vi "Matr_lin.vi"(2 "Date":u8, 3 "Linia":u8, 4 "Adresa port paralel":u16) -> (0 "C0-C3":u8, 1 "D0-D7":u8)   [LabVIEW 2009]
uses:
  <vilib>/Platform/portaccess.llb/Out Port8.vi
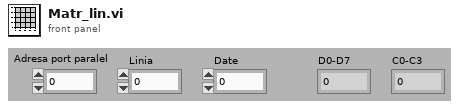
[diagram p1: front panel]
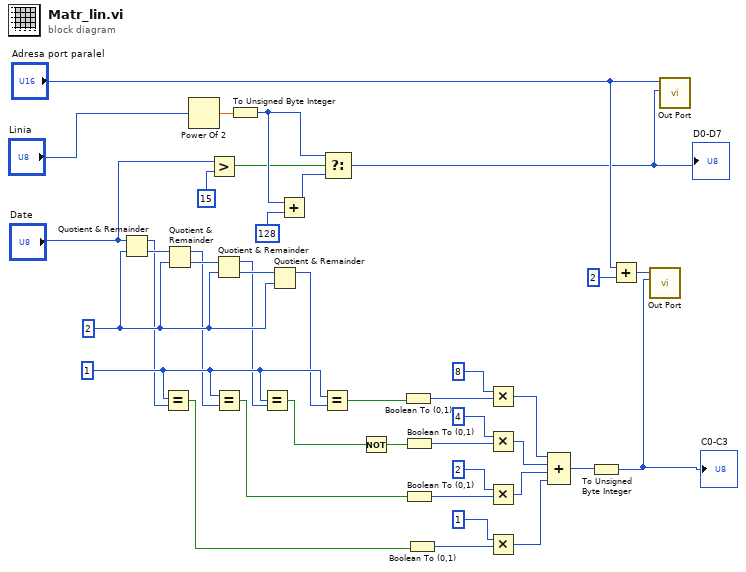
[diagram p0: block diagram]
diagram:
  w19 = 2
  w23 = 1
  n1 = Quotient & Remainder(x="Date", y=w19) -> (x-y*floor(x/y)=w15:i32, floor(x/y)=w22:i32)
  n2 = Equal?(x=w23, y=w15) -> (x = y?=w3:bool)
  n3 = Quotient & Remainder(x=w22, y=w19) -> (x-y*floor(x/y)=w16:i32, floor(x/y)=w21:i32)
  n4 = Power Of 2(x="Linia") -> (2^x=w13:dbl)
  n5 = Greater?(x="Date", y=u8 15) -> (0:w12:bool)
  n6 = Quotient & Remainder(x=w21, y=w19) -> (x-y*floor(x/y)=w17:i32, floor(x/y)=w20:i32)
  n7 = Equal?(x=w23, y=w16) -> (x = y?=w4:bool)
  n8 = To Unsigned Byte Integer(number=w13) -> (unsigned 8bit integer=w14:u8)
  n9 = Equal?(x=w23, y=w17) -> (x = y?=w1:bool)
  n10 = Quotient & Remainder(x=w20, y=w19) -> (x-y*floor(x/y)=w18:i32)  [unwired: 1 out]
  n11 = Add(x=w14, y=u8 128) -> (x+y=w10:u8)
  n12 = Equal?(x=w23, y=w18) -> (x = y?=w5:bool)
  n13 = Select(t=w14, s=w12, f=w10) -> (s? t:f=w37:u8)
  "D0-D7" <- w37
  n14 = Not(x=w1) -> (.not. x?=w2:bool)
  n15 = Boolean To (0,1)(Boolean=w5) -> (0, 1=w24:i16)
  n16 = Boolean To (0,1)(Boolean=w2) -> (0, 1=w26:i16)
  n17 = Boolean To (0,1)(Boolean=w4) -> (0, 1=w28:i16)
  n18 = Boolean To (0,1)(Boolean=w3) -> (0, 1=w32:i16)
  n19 = Multiply(x=8, y=w24) -> (x*y=w35:i32)
  n20 = Multiply(x=4, y=w26) -> (x*y=w30:i32)
  n21 = Multiply(x=2, y=w28) -> (x*y=w31:i32)
  n22 = Multiply(x=1, y=w32) -> (x*y=w34:i32)
  n23 = Compound Arithmetic op=ADD(w35, w30, w31, w34) -> (w36:i32)
  n24 = To Unsigned Byte Integer(number=w36) -> (unsigned 8bit integer=w38:u8)
  "C0-C3" <- w38
  n25 = Add(x="Adresa port paralel", y=u8 2) -> (x+y=w8:u16)
  n26 = call-poly <vilib>:"Out Port.vi"("write value"=w38, "address"=w8) -> ()  [unwired: 7 in, 1 out]
  n27 = call-poly <vilib>:"Out Port.vi"("write value"=w37, "address"="Adresa port paralel") -> ()  [unwired: 7 in, 1 out]
